vi "Run Centroid Detection.vi"(1 "Detection Parameters":T1) -> (0 "Run Detection":bool)   [LabVIEW 2013]
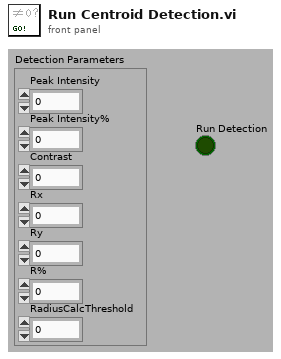
[diagram p1: front panel]
types:
  T1 = cluster{"Peak Intensity":i32, "Peak Intensity%":u8, "Contrast":i32, "Rx":sgl, "Ry":sgl, "R%":sgl, "RadiusCalcThreshold":u8}
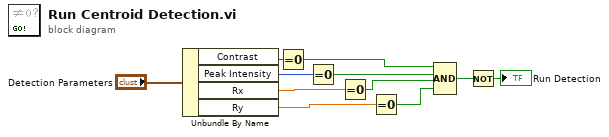
[diagram p0: block diagram]
diagram:
  n1 = Unbundle By Name("Detection Parameters") -> ("Contrast"=w10:i32, "Peak Intensity"=w9:i32, "Rx"=w8:sgl, "Ry"=w7:sgl)
  n2 = Equal To 0?(x=w10) -> (x = 0?=w6:bool)
  n3 = Equal To 0?(x=w9) -> (x = 0?=w5:bool)
  n4 = Equal To 0?(x=w8) -> (x = 0?=w4:bool)
  n5 = Equal To 0?(x=w7) -> (x = 0?=w3:bool)
  n6 = Compound Arithmetic op=AND(w6, w5, w4, w3) -> (w2:bool)
  n7 = Not(x=w2) -> (.not. x?=→"Run Detection":bool)
